vi "Replace Property Value.vi"(8 "error in (no error)":errorcluster, 9 "Property Type":i32(ring)=9 items=["K_STRING", "K_BOOL", "K_I32", "K_U32", "K_DOUBLE", "K_U64", "K_VARIANT", "K_DEPENDENTFILE", "K_DEPENDENTNODE", "K_DATASOURCENODE", "K_U16", "K_DBLARR", "K_U32ARR", "K_I32ARR", "K_STRINGARR", "K_DICTIONARY", "K_DICTIONARYARR", "K_BINARYSTRING", "K_I16", "K_I64", "K_BOOLARR", "K_U64ARR", "K_U16ARR", "K_I64ARR", "K_I16ARR"], 10 "Replacement Channels":T1={"Channel to Replace"="Targets/Controller/Custom Devices/VCOM/CAN_Sender_Tx/ACC/ACC_ESP_E2E_PR2/ACC_NEW_SIGNAL", "Replacement Channel"="Targets/Controller/User Channels/User Channel 1"}, 11 "NodeID":u64) -> (0 "error out":errorcluster, 3 "Replacement Log":string[](array[string]))   [LabVIEW 2025]
uses:
  Replacement Channels.ctl
  NationalInstruments.VeriStand.SystemStorage
  <vilib>/NI/NI VeriStand Advanced SysDef API/SysDef API/Advanced System Definition.lvlib
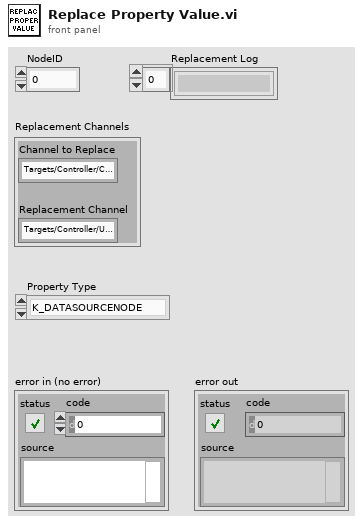
[diagram p1: front panel]
types:
  T1 = typedef "Replacement Channels.ctl" = cluster{"Channel to Replace":string, "Replacement Channel":string}
  T2 = typedef "Custom Device API.lvlib/Custom Device Pointer.ctl" = refnum<k24>
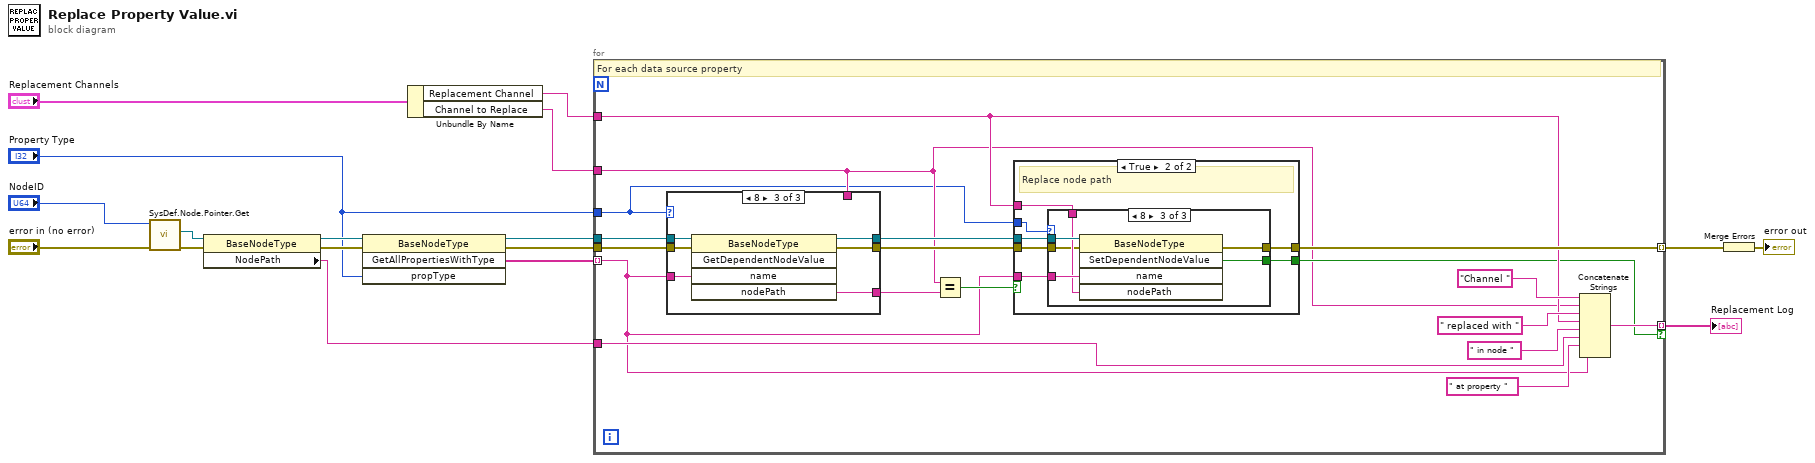
[diagram p0: block diagram]
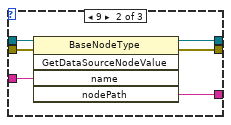
[diagram p3: hidden frame]
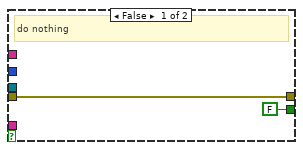
[diagram p4: hidden frame]
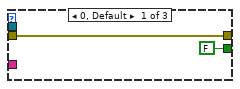
[diagram p5: hidden frame]
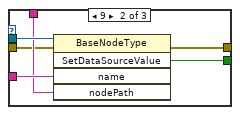
[diagram p6: hidden frame]
diagram:
  n1 = call <vilib>:"SysDef.Node.Pointer.Get.vi"("error in (no error)"="error in (no error)", "nodeID"="NodeID") -> ("error out"=w6:errorcluster, "Node Pointer"=w7:T2)  [unwired: 6 in, 2 out]
  n2 = property class="BaseNodeType"(reference=w7, error in=w6) -> (reference out=w5:T2, error out=w4:errorcluster, "NodePath"=w3:string)
  n3 = invoke class="BaseNodeType" method="GetAllPropertiesWithType"(reference=w5, error in=w4, "propType"="Property Type") -> (reference out=w8:T2, error out=w14:errorcluster, "GetAllPropertiesWithType"=w17:string[])  [unwired: 1 in, 1 out]
  n4 = Unbundle By Name("Replacement Channels") -> ("Replacement Channel"=w10:string, "Channel to Replace"=w9:string)
  n5 = for {
    tunnel: w8 -> [w35]
    tunnel: w17 -> [w22] mode=indexing
    tunnel: w9 -> [w19]
    tunnel: w10 -> [w26]
    tunnel: w14 -> [w31]
    tunnel: [w29] -> w13 mode=indexing
    tunnel: w3 -> [w24]
    tunnel: [w21] -> w2 mode=indexing if=w20
    tunnel: "Property Type" -> [w18]
    # "For each data source property"
    n6 = case shown="8" w18 {
      tunnel: w35 -> [w38 w44 w50]
      tunnel: [w38 w43 w49] -> w34
      tunnel: [w36 w42 w48] -> w33
      tunnel: w31 -> [w37 w41 w47]
      tunnel: [w37 w40 w46] -> w30
      tunnel: w22 -> [_ w39 w45]
      tunnel: w19 -> [w36 _ _]
      frame 0, Default {
      }
      frame 9 {
        n7 = invoke class="BaseNodeType" method="GetDataSourceNodeValue"(reference=w44, error in=w41, "name"=w39) -> (reference out=w43:T2, error out=w40:errorcluster, "nodePath"=w42:string)  [unwired: 2 in, 2 out]
      }
      frame 8 {
        n8 = invoke class="BaseNodeType" method="GetDependentNodeValue"(reference=w50, error in=w47, "name"=w45) -> (reference out=w49:T2, error out=w46:errorcluster, "nodePath"=w48:string)  [unwired: 2 in, 2 out]
      }
    }
    n9 = Equal?(x=w19, y=w33) -> (x = y?=w32:bool)
    n10 = case shown="True" w32 {
      tunnel: w34 -> [_ w59]
      tunnel: w22 -> [_ w58]
      tunnel: w26 -> [_ w57]
      tunnel: w30 -> [w52 w56]
      tunnel: [w52 w55] -> w29
      tunnel: [FALSE ("SetDataSourceValue") w54] -> w20
      tunnel: w18 -> [_ w53]
      frame False {
        # "do nothing"
      }
      frame True {
        # "Replace node path"
        n11 = case shown="8" w53 {
          tunnel: w59 -> [_ w67 w73]
          tunnel: w58 -> [_ w66 w72]
          tunnel: w57 -> [_ w65 w71]
          tunnel: w56 -> [w61 w64 w70]
          tunnel: [w61 w63 w69] -> w55
          tunnel: [FALSE ("SetDependentNodeValue") w62 w68] -> w54
          frame 0, Default {
          }
          frame 9 {
            n12 = invoke class="BaseNodeType" method="SetDataSourceValue"(reference=w67, error in=w64, "name"=w66, "nodePath"=w65) -> (error out=w63:errorcluster, "SetDataSourceValue"=w62:bool)  [unwired: 1 in, 3 out]
          }
          frame 8 {
            n13 = invoke class="BaseNodeType" method="SetDependentNodeValue"(reference=w73, error in=w70, "name"=w72, "nodePath"=w71) -> (error out=w69:errorcluster, "SetDependentNodeValue"=w68:bool)  [unwired: 1 in, 3 out]
          }
        }
      }
    }
    n14 = Concatenate Strings("Channel " ("string"), w19, " replaced with " ("string"), w26, " in node " ("string"), w24, " at property " ("string"), w22) -> (w21:string)
  }
  "Replacement Log" <- w2
  n15 = Merge Errors(w13) -> (→"error out":errorcluster)
